vi "FindSimETH.vi"(6 "COM":string, 8 "error in (no error)":errorcluster) -> (0 "error out":errorcluster, 1 "Pass":bool, 2 "CmdOut":string)   [LabVIEW 2013]
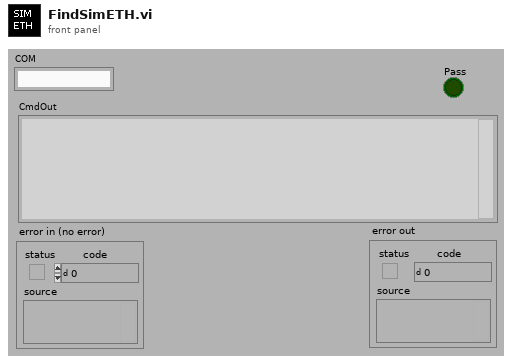
[diagram p1: front panel]
types:
  T1 = enum32{"invalid app kind", "Development System", "Run Time System", "Student Edition", "Embedded LabVIEW", "Evaluation", "Custom"}
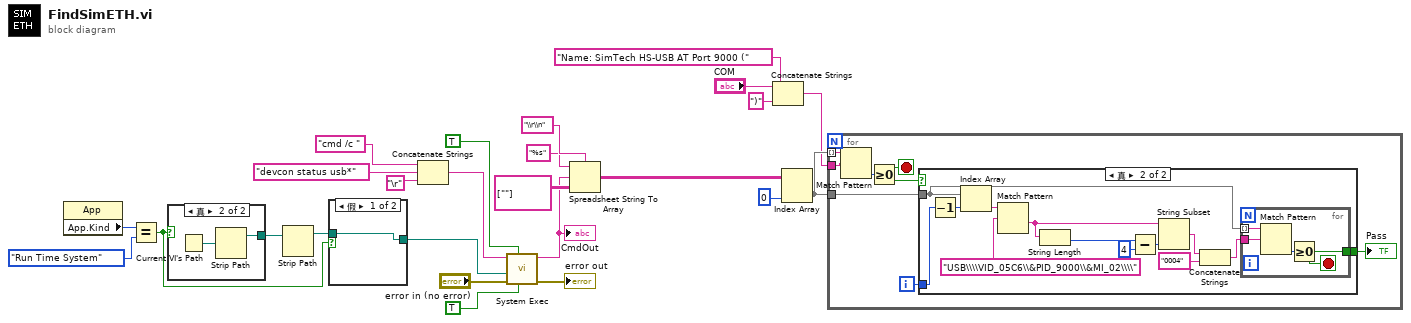
[diagram p0: block diagram]
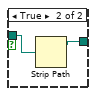
[diagram p2: hidden frame]
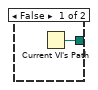
[diagram p3: hidden frame]
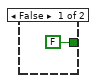
[diagram p4: hidden frame]
diagram:
  n1 = property class="App"() -> ("App.Kind"=w12:T1)  [unwired: 2 in, 2 out]
  n2 = Equal?(x=w12, y=T1."Run Time System") -> (x = y?=w1:bool)
  n3 = case shown="真" w1 {
    tunnel: [w26 w28] -> w11
    frame False {
      n4 = Current VI's Path() -> (path=w26:path)
    }
    frame True {
      n5 = Current VI's Path() -> (path=w27:path)
      n6 = Strip Path(path=w27) -> (stripped path=w28:path)  [unwired: 1 out]
    }
  }
  n7 = Strip Path(path=w11) -> (stripped path=w3:path)  [unwired: 1 out]
  n8 = case shown="假" w1 {
    tunnel: w3 -> [w29 w31]
    tunnel: [w29 w30] -> w2
    frame False {
    }
    frame True {
      n9 = Strip Path(path=w31) -> (stripped path=w30:path)  [unwired: 1 out]
    }
  }
  n10 = Concatenate Strings("cmd /c " ("command line"), "devcon status usb*" ("command"), "\r") -> (w23:string)
  n11 = call <vilib>:"System Exec.vi"("run minimized? (F)"=TRUE, "wait until completion? (T)"=TRUE, "error in (no error)"="error in (no error)", "working directory"=w2, "command line"=w23) -> ("error out"=→"error out":errorcluster, "standard output"=w14:string)  [unwired: 1 in, 4 out]
  "CmdOut" <- w14
  n12 = Spreadsheet String To Array(delimiter (Tab)="\\r\\n" ("格式字符串"), format string="%s" ("格式字符串"), spreadsheet string=w14, array type (2D Dbl)=string[][] [[""]]) -> (array=w16:string[][])
  n13 = Concatenate Strings("Name: SimTech HS-USB AT Port 9000 (" ("command line"), "COM", ")" ("字符串")) -> (w5:string)
  n14 = Index Array(array=w16, index (col)=0 ("索引 (行)")) -> (element=w8:string[])  [unwired: 1 in]
  n15 = for {
    tunnel: w8 -> [w38] mode=indexing
    tunnel: w5 -> [w37]
    tunnel: w8 -> [w35]
    i -> [w36]
    stop <- w33 stop-if-true
    n16 = Match Pattern(string=w38, regular expression=w37) -> (offset past match=w34:i32)  [unwired: 4 out]
    n17 = Greater Or Equal To 0?(x=w34) -> (x >= 0?=w33:bool)
    n18 = case shown="真" w33 {
      tunnel: w36 -> [_ w52]
      tunnel: w35 -> [_ w42]
      tunnel: [FALSE w40] -> w32
      frame False {
      }
      frame True {
        n19 = Decrement(x=w52) -> (x-1=w51:i32)
        n20 = Index Array(array=w42, index=w51) -> (element=w45:string)
        n21 = Match Pattern(string=w45, regular expression="USB\\\\VID_05C6\\&PID_9000\\&MI_02\\\\" ("正则表达式")) -> (after substring=w49:string)  [unwired: 1 in, 3 out]
        n22 = String Length(string=w49) -> (length=w48:i32)
        n23 = Subtract(x=w48, y=4) -> (x-y=w46:i32)
        n24 = String Subset(string=w49, length (rest)=w46) -> (substring=w43:string)  [unwired: 1 in]
        n25 = Concatenate Strings(w43, "0004" ("字符串")) -> (w41:string)
        n26 = for {
          tunnel: w42 -> [w56] mode=indexing
          tunnel: [w54] -> w40
          tunnel: w41 -> [w53]
          stop <- w54 stop-if-true
          n27 = Match Pattern(string=w56, regular expression=w53) -> (offset past match=w55:i32)  [unwired: 1 in, 3 out]
          n28 = Greater Or Equal To 0?(x=w55) -> (x >= 0?=w54:bool)
        }
      }
    }
    "Pass" <- w32
  }
